vi "Test Display_HE.vi"(0 "Expected LEDs":T7, 5 "Care?":T8, 7 "Actual LEDs":T7, 11 "error in":errorcluster) -> (4 "Pass/Fail?":bool, 6 "Report Text":string, 15 "error out":errorcluster)   [LabVIEW 2016, in "Centauro.lvlib"]
uses:
  Projects/Centauro.lvlib
  controls/HEUI_Display.ctl
  controls/HEUI_Display_Care.ctl
  controls/Cycle Selection Enum.ctl
  controls/Stain Enum.ctl
  controls/Temp Enum.ctl
  controls/Soil Enum.ctl
  controls/Spin Enum.ctl
  controls/750 Status Enum.ctl
panel:
  in  "Spin Level":T1
  in  "eMonitor Level":T2
  in  "Soil Level":T3
  in  "Temp Level":T4
  in  "Stain Selection":T5
  in  "Cycle Selection":T6
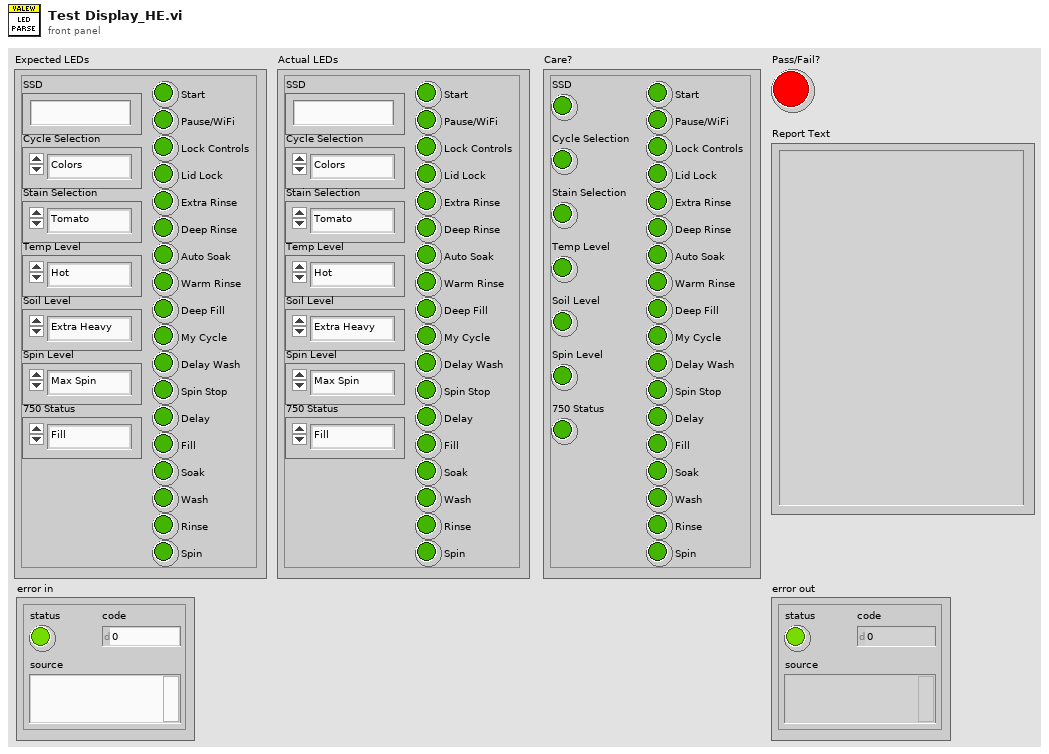
[diagram p1: front panel]
types:
  T1 = typedef "Centauro.lvlib/Spin Enum.ctl" = enum16{"Max Spin", "More Spin", "Normal Spin", "No Spin", "Off", "*Incorrect*"}
  T2 = typedef "Centauro.lvlib/750 Status Enum.ctl" = enum16{"Fill", "Wash", "Rinse", "Spin", "Off", "*Incorrect*"}
  T3 = typedef "Centauro.lvlib/Soil Enum.ctl" = enum16{"Extra Heavy", "Heavy", "Normal", "Light", "Off", "*Incorrect*"}
  T4 = typedef "Centauro.lvlib/Temp Enum.ctl" = enum16{"Hot", "Warm", "Colors", "Cool", "Cold", "Tap Cold", "Off", "*Incorrect*"}
  T5 = typedef "Centauro.lvlib/Stain Enum.ctl" = enum16{"Tomato", "Wine", "Blood", "Grass", "Dirt", "Off", "*Incorrect*"}
  T6 = typedef "Centauro.lvlib/Cycle Selection Enum.ctl" = enum16{"Colors", "Easy Care", "Delicates", "Hand Wash", "Active Wear", "Speed Wash", "Rinse and Spin", "Drain and Spin", "Basket Clean", "Jeans", "Heavy Duty", "Bulky Items", "Towels", "Whites", "Off", "*Incorrect*"}
  T7 = typedef "Centauro.lvlib/HEUI_Display.ctl" = cluster{"SSD":string, "Cycle Selection":T6, "Stain Selection":T5, "Temp Level":T4, "Soil Level":T3, "Spin Level":T1, "750 Status":T2, "Start":bool, "Pause/WiFi":bool, "Lock Controls":bool, "Lid Lock":bool, "Extra Rinse":bool, "Deep Rinse":bool, "Auto Soak":bool, "Warm Rinse":bool, "Deep Fill":bool, "My Cycle":bool, "Delay Wash":bool, "Spin Stop":bool, "Delay":bool, "Fill":bool, "Soak":bool, "Wash":bool, "Rinse":bool, "Spin":bool}
  T8 = typedef "Centauro.lvlib/HEUI_Display_Care.ctl" = cluster{"SSD":bool, "Cycle Selection":bool, "Stain Selection":bool, "Temp Level":bool, "Soil Level":bool, "Spin Level":bool, "750 Status":bool, "Start":bool, "Pause/WiFi":bool, "Lock Controls":bool, "Lid Lock":bool, "Extra Rinse":bool, "Deep Rinse":bool, "Auto Soak":bool, "Warm Rinse":bool, "Deep Fill":bool, "My Cycle":bool, "Delay Wash":bool, "Spin Stop":bool, "Delay":bool, "Fill":bool, "Soak":bool, "Wash":bool, "Rinse":bool, "Spin":bool}
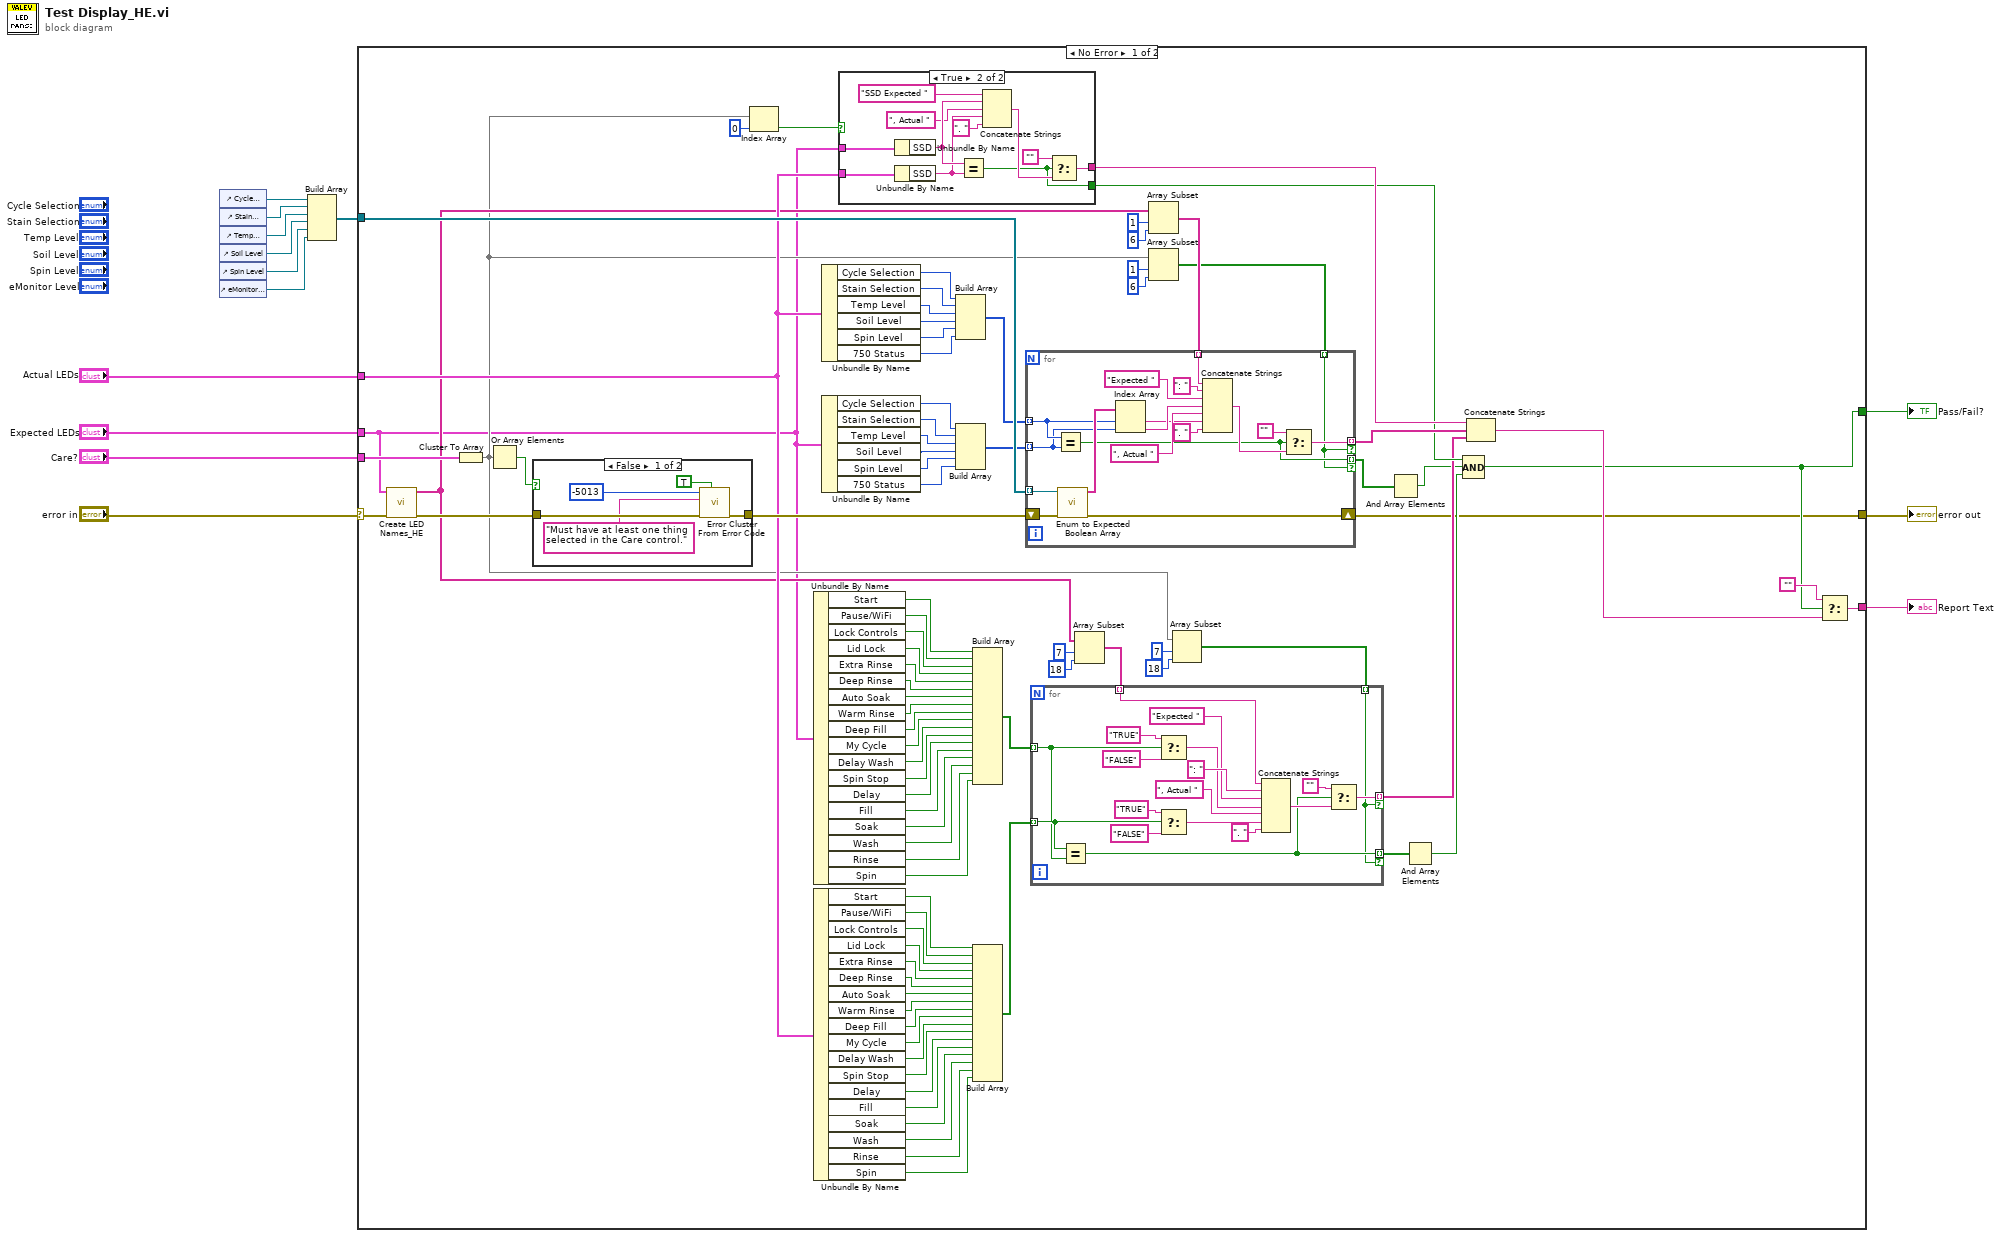
[diagram p0: block diagram]
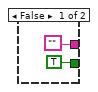
[diagram p2: hidden frame]
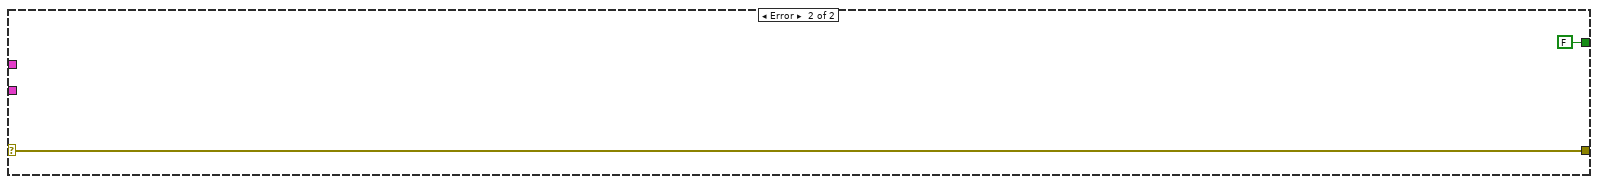
[diagram p4: hidden frame]
diagram:
  n1 = control-ref of="Cycle Selection"() -> (w1:refnum<vi>)
  n2 = control-ref of="Stain Selection"() -> (w2:refnum<vi>)
  n3 = control-ref of="Temp Level"() -> (w7:refnum<vi>)
  n4 = control-ref of="Soil Level"() -> (w6:refnum<vi>)
  n5 = control-ref of="Spin Level"() -> (w5:refnum<vi>)
  n6 = control-ref of="eMonitor Level"() -> (w4:refnum<vi>)
  n7 = Build Array(w1, w2, w7, w6, w5, w4) -> (w3:refnum<vi>[])
  n8 = case shown="No Error" "error in" {
    selector: "error in" -> [w101 w160]
    tunnel: [w35 w160] -> w14
    tunnel: [w102 _] -> w13
    tunnel: "Care?" -> [w99 _]
    tunnel: "Expected LEDs" -> [w17 _]
    tunnel: "Actual LEDs" -> [w54 _]
    tunnel: [w36 FALSE] -> w8
    tunnel: w3 -> [w93 _]
    frame No Error {
      n9 = call "Create LED Names_HE.vi"("Expected LEDs"=w17, "Error In"=w101) -> ("Array of LED Names"=w45:string[], "Error Out"=w98:errorcluster)  [unwired: 12 in]
      n10 = Cluster To Array(cluster=w99) -> (array=w18:bool[])
      n11 = Or Array Elements(Boolean array=w18) -> (logical OR=w100:bool)
      n12 = case shown="False" w100 {
        tunnel: w98 -> [w157 w158]
        tunnel: [w156 w158] -> w82
        frame False {
          n13 = call <vilib>:"Error Cluster From Error Code.vi"("show call chain? (False)"=TRUE, "error in (no error)"=w157, "error message (\"\")"="Must have at least one thing selected in the Care control." ("error message (\"\")"), "error code (0)"=-5013) -> ("error out"=w156:errorcluster)  [unwired: 5 in]
        }
        frame True {
        }
      }
      n14 = Index Array(array=w18, index=0) -> (element=w51:bool)
      n15 = Unbundle By Name(w17) -> ("Start"=w68:bool, "Pause/WiFi"=w67:bool, "Lock Controls"=w66:bool, "Lid Lock"=w65:bool, "Extra Rinse"=w64:bool, "Deep Rinse"=w63:bool, "Auto Soak"=w62:bool, "Warm Rinse"=w61:bool, "Deep Fill"=w60:bool, "My Cycle"=w59:bool, "Delay Wash"=w58:bool, "Spin Stop"=w57:bool, "Delay"=w30:bool, "Fill"=w29:bool, "Soak"=w28:bool, "Wash"=w27:bool, "Rinse"=w26:bool, "Spin"=w25:bool)
      n16 = Unbundle By Name(w54) -> ("Start"=w80:bool, "Pause/WiFi"=w79:bool, "Lock Controls"=w78:bool, "Lid Lock"=w77:bool, "Extra Rinse"=w76:bool, "Deep Rinse"=w75:bool, "Auto Soak"=w74:bool, "Warm Rinse"=w73:bool, "Deep Fill"=w72:bool, "My Cycle"=w71:bool, "Delay Wash"=w70:bool, "Spin Stop"=w69:bool, "Delay"=w24:bool, "Fill"=w23:bool, "Soak"=w22:bool, "Wash"=w21:bool, "Rinse"=w20:bool, "Spin"=w19:bool)
      n17 = Unbundle By Name(w54) -> ("Cycle Selection"=w33:T6, "Stain Selection"=w34:T5, "Temp Level"=w97:T4, "Soil Level"=w96:T3, "Spin Level"=w95:T1, "750 Status"=w94:T2)
      n18 = Unbundle By Name(w17) -> ("Cycle Selection"=w31:T6, "Stain Selection"=w32:T5, "Temp Level"=w85:T4, "Soil Level"=w86:T3, "Spin Level"=w87:T1, "750 Status"=w88:T2)
      n19 = case shown="True" w51 {
        tunnel: ["" w127] -> w81
        tunnel: w54 -> [_ w126]
        tunnel: w17 -> [_ w125]
        tunnel: [TRUE w124] -> w53
        frame False {
        }
        frame True {
          n20 = Unbundle By Name(w125) -> ("SSD"=w132:string)
          n21 = Unbundle By Name(w126) -> ("SSD"=w130:string)
          n22 = Equal?(x=w132, y=w130) -> (x = y?=w124:bool)
          n23 = Concatenate Strings("SSD Expected " ("string"), w132, ", Actual " ("string"), w130, ". " ("string")) -> (w128:string)
          n24 = Select(t="", s=w124, f=w128) -> (s? t:f=w127:string)
        }
      }
      n25 = Build Array(w33, w34, w97, w96, w95, w94) -> (w92:u16[])
      n26 = Build Array(w31, w32, w85, w86, w87, w88) -> (w84:u16[])
      n27 = Build Array(w68, w67, w66, w65, w64, w63, w62, w61, w60, w59, w58, w57, w30, w29, w28, w27, w26, w25) -> (w49:bool[])
      n28 = Build Array(w80, w79, w78, w77, w76, w75, w74, w73, w72, w71, w70, w69, w24, w23, w22, w21, w20, w19) -> (w50:bool[])
      n29 = Array Subset(array=w45, index=7, length=18) -> (w46:string[])
      n30 = Array Subset(array=w45, index=1, length=6) -> (w89:string[])
      n31 = Array Subset(array=w18, index=1, length=6) -> (w15:bool[])
      n32 = for {
        tunnel: w93 -> [w152] mode=indexing
        shift-right: [w150] -> w35
        shift-left: w82 -> [w151]
        tunnel: w92 -> [w147] mode=indexing
        tunnel: w84 -> [w146] mode=indexing
        tunnel: w89 -> [w145] mode=indexing
        tunnel: [w137] -> w83 mode=indexing if=w135
        tunnel: [w136] -> w39 mode=indexing if=w135
        tunnel: w15 -> [w135] mode=indexing
        n33 = Equal?(x=w147, y=w146) -> (x = y?=w136:bool)
        n34 = call "Enum to Expected Boolean Array.vi"("reference"=w152, "error in (no error)"=w151) -> ("Enum Names"=w148:string[], "error out"=w150:errorcluster)  [unwired: 11 in, 1 out]
        n35 = Index Array(array=w148, index #1=w147, index #2=w146) -> (element #1=w140:string, element #2=w142:string)
        n36 = Concatenate Strings(w145, ": " ("string"), "Expected " ("string"), w142, ", Actual " ("string"), w140, ". " ("string")) -> (w138:string)
        n37 = Select(t="", s=w136, f=w138) -> (s? t:f=w137:string)
      }
      n38 = Array Subset(array=w18, index=7, length=18) -> (w16:bool[])
      n39 = for {
        tunnel: w50 -> [w112] mode=indexing
        tunnel: w49 -> [w106] mode=indexing
        tunnel: [w115] -> w42 mode=indexing if=w113
        tunnel: [w114] -> w38 mode=indexing if=w113
        tunnel: w16 -> [w113] mode=indexing
        tunnel: w46 -> [w104] mode=indexing
        n40 = Equal?(x=w112, y=w106) -> (x = y?=w114:bool)
        n41 = Select(t="TRUE" ("string"), s=w106, f="FALSE" ("string")) -> (s? t:f=w105:string)
        n42 = Select(t="TRUE" ("string"), s=w112, f="FALSE" ("string")) -> (s? t:f=w109:string)
        n43 = Concatenate Strings(w104, ": " ("string"), "Expected " ("string"), w105, ", Actual " ("string"), w109, ". " ("string")) -> (w116:string)
        n44 = Select(t="", s=w114, f=w116) -> (s? t:f=w115:string)
      }
      n45 = And Array Elements(Boolean array=w39) -> (logical AND=w40:bool)
      n46 = And Array Elements(Boolean array=w38) -> (logical AND=w37:bool)
      n47 = Compound Arithmetic op=AND(w53, w40, w37) -> (w36:bool)
      n48 = Concatenate Strings(w81, w83, w42) -> (w41:string)
      n49 = Select(t="", s=w36, f=w41) -> (s? t:f=w102:string)
    }
    frame Error {
    }
  }
  "error out" <- w14
  "Pass/Fail?" <- w8
  "Report Text" <- w13
